vi "Input Device Module.vi"(7 "This VI":refnum<vi>, 9 "Movables Channel in":T1, 10 "Communication in":refnum<class "Communication.lvclass">, 11 "Game Settings in":T2 {"FPS" items=["120"=8, "60"=16]; "Difficulty" items=["Hard"=1.0, "Medium"=0.9, "Easy"=0.8]; "Players Number" items=["2"=2, "4"=4]}) -> (0 "error out":errorcluster)   [LabVIEW 2024, in "Input Device.lvclass"]
uses:
  Input Device.lvclass
  Communication/Communication.lvclass
  Type Def/Game Settings.ctl
  Type Def/Control Device.ctl
  Type Def/Players Number.ctl
  Type Def/Difficulty.ctl
  Type Def/FPS.ctl
  Type Def/Mode.ctl
  <extravilib>/ChannelInstances/Tag-a[.](class'Movable')/))Channel.ctl
  Game Componants/Game Board Component/Movable/Movable.lvclass
  C:/Users/David/Documents/Project/2D Game LabVIEW/The-LabVIEW-Soccer-Game/Source/Game Componants/Game Componants.lvclass
  Keyboard/Keyboard.lvclass
  C:/Users/David/Documents/Project/2D Game LabVIEW/The-LabVIEW-Soccer-Game/Source/Input Device/Input Device.lvclass
  Xbox Controller/Xbox Controller.lvclass
  Mouse/Mouse.lvclass
  Communication/Communication.lvclass/Communication.ctl
  Game Componants/Game Componants.lvclass/Game Componants.ctl
  Mouse/Mouse.lvclass/Mouse.ctl
  <extravilib>/ChannelInstances/Tag-a[.](class'Movable')/Read With Abort.vi
  <extravilib>/ChannelInstances/Tag-a[.](class'Movable')/EndpointRead.vi
  Game Componants/Game Componants.lvclass
  <extravilib>/ChannelInstances/Tag-a[.](class'Movable').lvlib
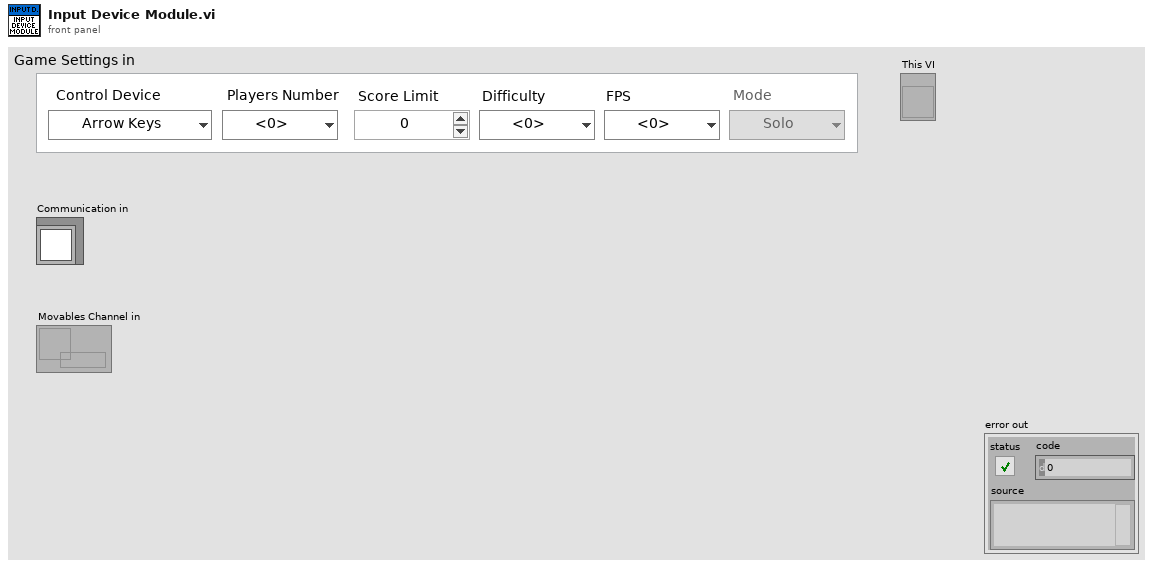
[diagram p1: front panel]
types:
  T1 = typedef "Tag-a[.](class'Movable').lvlib/))Channel.ctl" = refnum<queue>
  T2 = typedef "Game Settings.ctl" = cluster{"Control Device":T3, "Players Number":T4, "Score Limit":u8, "Difficulty":T5, "FPS":T6, "Mode":T7, "Player ID":u8}
  T3 = typedef "Control Device.ctl" = enum16{"Arrow Keys", "Mouse", "Xbox Controller"}
  T4 = typedef "Players Number.ctl" = u16
  T5 = typedef "Difficulty.ctl" = dbl
  T6 = typedef "FPS.ctl" = u8
  T7 = typedef "Mode.ctl" = enum16{"Solo", "Multiplayer"}
  T8 = typedef "Coordinates.ctl" = cluster{"x":dbl, "y":dbl}
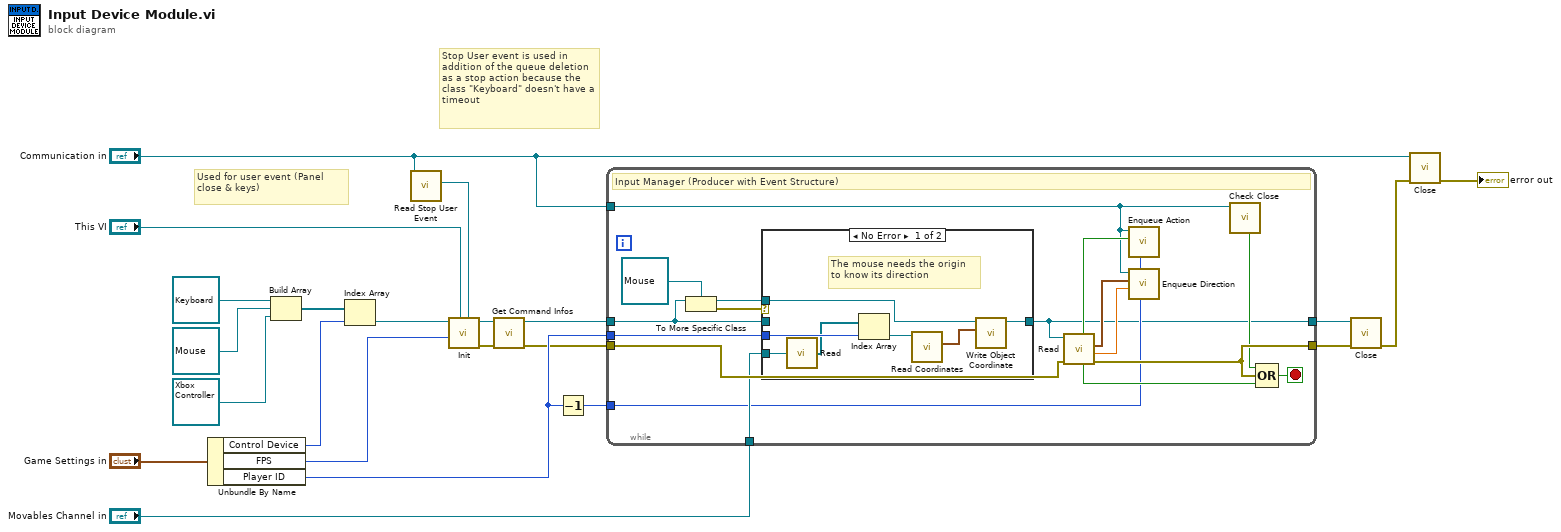
[diagram p0: block diagram]
diagram:
  # "Used for user event (Panel close & keys)"
  # "Stop User event is used in addition of the queue deletion as a stop action because the class \"Keyboard\" doesn't have a timeout"
  n1 = Unbundle By Name("Game Settings in") -> ("Control Device"=w20:T3, "FPS"=w21:T6, "Player ID"=w19:u8)
  n2 = Build Array(refnum<class "Keyboard.lvclass"> refnum ("Keyboard.lvclass"), refnum<class "Mouse.lvclass"> refnum ("Mouse.lvclass"), refnum<class "Xbox Controller.lvclass"> refnum ("Xbox Controller.lvclass")) -> (w12:refnum<class "Input Device.lvclass">[])
  n3 = Index Array(array=w12, index=w20) -> (element=w13:refnum<class "Input Device.lvclass">)
  n4 = call "Read Stop User Event.vi"("Communication in"="Communication in") -> ("Stop User Event"=w2:refnum<user-event>)  [unwired: 10 in]
  n5 = call-dynamic "Init.vi"("Stop User Event in"=w2, "Ref FP in"="This VI", "Period (ms) in"=w21, "Input Device in"=w13) -> ("error out"=w3:errorcluster, "Input Device out"=w6:refnum<class "Input Device.lvclass">)  [unwired: 6 in]
  n6 = call-dynamic "Get Command Infos.vi"("error in (no error)"=w3, "Input Device in"=w6) -> ("error out"=w5:errorcluster, "Input Device out"=w7:refnum<class "Input Device.lvclass">)  [unwired: 6 in, 2 out]
  n7 = Decrement(x=w19) -> (x-1=w16:u8)
  n8 = while {
    tunnel: w5 -> [w32]
    tunnel: w7 -> [w34]
    tunnel: [w39] -> w15
    tunnel: w19 -> [w31]
    tunnel: "Movables Channel in" -> [w30]
    tunnel: "Communication in" -> [w28]
    tunnel: w16 -> [w24]
    tunnel: [w23] -> w1
    stop <- w37 stop-if-true
    # "Input Manager (Producer with Event Structure)"
    n9 = To More Specific Class(target class=refnum<class "Mouse.lvclass"> refnum ("Mouse.lvclass"), reference=w34) -> (specific class reference=w33:refnum<class "Mouse.lvclass">, error out=w35:errorcluster)  [unwired: 1 in]
    n10 = case shown="No Error" w35 {
      tunnel: w34 -> [_ w47]
      tunnel: [w45 w47] -> w23
      tunnel: w33 -> [w46 _]
      tunnel: w31 -> [w44 _]
      tunnel: w30 -> [w41 _]
      frame No Error {
        # "The mouse needs the origin to know its direction"
        n11 = call <extravilib>:"Read.vi"("channel"=w41) -> ("element"=w40:refnum<class "Movable.lvclass">[])  [unwired: 1 in, 1 out]
        n12 = Index Array(array=w40, index=w44) -> (element=w43:refnum<class "Movable.lvclass">)
        n13 = call "Read Coordinates.vi"("Game Componants in"=w43) -> ("Coordinates"=w42:T8)  [unwired: 10 in]
        n14 = call "Write Object Coordinate.vi"("Object Coordinate"=w42, "Mouse in"=w46) -> ("Mouse out"=w45:refnum<class "Mouse.lvclass">)  [unwired: 9 in]
      }
      frame Error {
      }
    }
    n15 = call-dynamic <extravilib>:"Read.vi"("error in (no error)"=w32, "Input Device in"=w23) -> ("error out"=w39:errorcluster, "Velocity out"=w26:dbl, "Direction out"=w27:cluster{dbl, dbl}, "Stop?"=w38:bool, "Boost?"=w29:bool)  [unwired: 5 in]
    n16 = call "Enqueue Action.vi"("Index in"=w24, "Boost in"=w29, "Communication in"=w28) -> ()  [unwired: 9 in]
    n17 = call "Enqueue Direction.vi"("Index in"=w24, "Velocity in"=w26, "Direction in"=w27, "Communication in"=w28) -> ()  [unwired: 8 in]
    n18 = call "Check Close.vi"("Communication in"=w28) -> ("Stop?"=w25:bool)  [unwired: 10 in]
    n19 = Compound Arithmetic op=OR(w25, w39, w38) -> (w37:bool)
  }
  n20 = call-dynamic "Close.vi"("error in (no error)"=w15, "Input Device in"=w1) -> ("error out"=w17:errorcluster)  [unwired: 9 in]
  n21 = call "Close.vi"("error in (no error)"=w17, "Communication in"="Communication in") -> ("error out"=→"error out":errorcluster)  [unwired: 9 in]
